vi "Begin.vi"(8 "error in":errorcluster) -> (0 "error out":errorcluster)   [LabVIEW 2020]
doc: "Called before other user functions, this VI is expected to open initial I/O refnums, load in file data, and do all program initialization. Notice that the <B>error out</B> terminal is simply used for data flow. Wiring it to other structures or subVIs ensures that this VI runs first."
uses:
  <vilib>/Rock Robotics/WPI/DriverStation/WPI_DriverStationRobotMode2.ctl
  <vilib>/Rock Robotics/WPI/Joystick/WPI_JoystickDeviceEnum.ctl
  <vilib>/Rock Robotics/SystemInterfaces/i2clib/i2c_bus.ctl
  <vilib>/Rock Robotics/SystemInterfaces/DIO/FPGA_DIOChannel.ctl
  Robot Global Data.vi
  <vilib>/Rock Robotics/Network Tables/NT Write String Array.vi
  <vilib>/Rock Robotics/WPI/ThirdParty/Phoenix-LabVIEW/Motor Controller/Get/CTRE_Phoenix_MotorController_GetSelectedSensorData.vi
  <vilib>/Rock Robotics/WPI/Switch/WPI_SwitchOpenLimit.vi
  <vilib>/Rock Robotics/WPI/Switch/WPI_SwitchOpenCounting.vi
  <vilib>/Rock Robotics/WPI/ThirdParty/Phoenix-LabVIEW/Motor Controller/Get/CTRE_Phoenix_MotorController_IntegratedSensorData_TalonFX.vi
  GlobalAutonVariables.vi
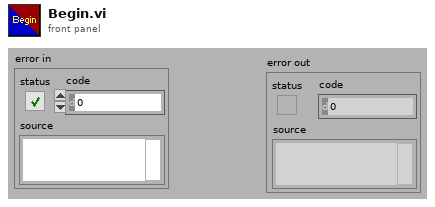
[diagram p1: front panel]
types:
  T1 = typedef "FPGA_DIOChannel.ctl" = enum8{"DIO 0", "DIO 1", "DIO 2", "DIO 3", "DIO 4", "DIO 5", "DIO 6", "DIO 7", "DIO 8", "DIO 9", "DIO MXP 0", "DIO MXP 1", "DIO MXP 2", "DIO MXP 3", "DIO MXP 4", "DIO MXP 5", "DIO MXP 6", "DIO MXP 7", "DIO MXP 8", "DIO MXP 9", "DIO MXP 10", "DIO MXP 11", "DIO MXP 12", "DIO MXP 13", "DIO MXP 14", "DIO MXP 15", "SPI Port CS1", "SPI Port CS2", "SPI Port CS3", "SPI Port MISO", "SPI Port MOSI", "Invalid"}
  T2 = typedef "i2c_bus.ctl" = enum16{"I2C On-Board", "I2C MXP", "Invalid"}
  T3 = typedef "WPI_JoystickDeviceEnum.ctl" = enum16{"USB 0", "USB 1", "USB 2", "USB 3", "USB 4", "USB 5"}
  T4 = typedef "WPI_DriverStationRobotMode2.ctl" = enum16{"Autonomous Disabled", "Autonomous Enabled", "Teleop Disabled", "Teleop Enabled", "Disconnected", "Finish", "Test Disabled", "Test Enabled", "Emergency Stopped"}
  T5 = typedef "WPI_CompressorDevRef.ctl" = cluster{"DevStatus":errorcluster, "Pneumatics Control Module":u8}
  T6 = typedef "WPI_JoystickDevRef.ctl" = cluster{"Device":T3}
  T7 = typedef "WPI_MotorControlDeviceRef.ctl" = cluster{"DeviceStatus":errorcluster, "Type":T8, "PWM":cluster{"PWM Channel":T9, "DeadBand":T10}, "CAN":cluster{"Device Number":u8, "SetOutput VI Ref":variant, "GetOutput VI Ref":variant, "Enable VI Ref":variant, "Disable VI Ref":variant, "Data":variant}, "Invert":bool, "DIO PWM":cluster{"PWM \"Enable\" Channel":T9, "DIOChannel":T1, "PWM Rate":dbl}}
  T8 = typedef "WPI_MotorControlType.ctl" = enum16{"PWM", "CAN", "DIO PWM"}
  T9 = typedef "FPGA_DIOPWMChannel.ctl" = enum8{"PWM 0", "PWM 1", "PWM 2", "PWM 3", "PWM 4", "PWM 5", "PWM 6", "PWM 7", "PWM 8", "PWM 9", "PWM MXP 0", "PWM MXP 1", "PWM MXP 2", "PWM MXP 3", "PWM MXP 4", "PWM MXP 5", "PWM MXP 6", "PWM MXP 7", "PWM MXP 8", "PWM MXP 9", "Invalid"}
  T10 = typedef "WPI_PWMDeadband.ctl" = cluster{"Name":string, "maxPositivePwm":i32, "minPositivePwm":i32, "centerPwm":i32, "maxNegativePwm":i32, "minNegativePwm":i32, "angularRange":u16}
  T11 = typedef "Color Sensor V3 DevRef.ctl" = cluster{"I2CDevRef":T12}
  T12 = typedef "WPI_I2CDevRef.ctl" = cluster{"DevStatus":errorcluster, "Device Address":u8, "Handle":i32, "I2C Bus":T2}
  T13 = typedef "CTRE_PigeonIMU_DeviceRef.ctl" = cluster{"DeviceStatus":errorcluster, "Device Number":u8, "Type":T14, "Device ID":u32, "Handle":u64, "UsageFrame":u32, "Library Path":path}
  T14 = typedef "CTRE_PigeonIMU_ConnectionType.ctl" = u32
  T15 = typedef "CTRE_Phoenix_CANcoder_DeviceRef.ctl" = cluster{"DeviceStatus":errorcluster, "Device Number":u8, "Handle":u64, "UsageFrame":u32, "Library Path":path}
  T16 = typedef "WPI_SwitchDevRef.ctl" = cluster{"DevStatus":errorcluster, "DIO Channel":T1, "CntIndex":T17, "Normally Closed":bool}
  T17 = typedef "FPGA_CounterCtrSystemIndex.ctl" = enum8{"Ctr 0", "Ctr 1", "Ctr 2", "Ctr 3", "Ctr 4", "Ctr 5", "Ctr 6", "Ctr 7", "Invalid"}
  T18 = enum16{"open", "replace", "create", "open or create", "replace or create", "replace or create with confirmation"}
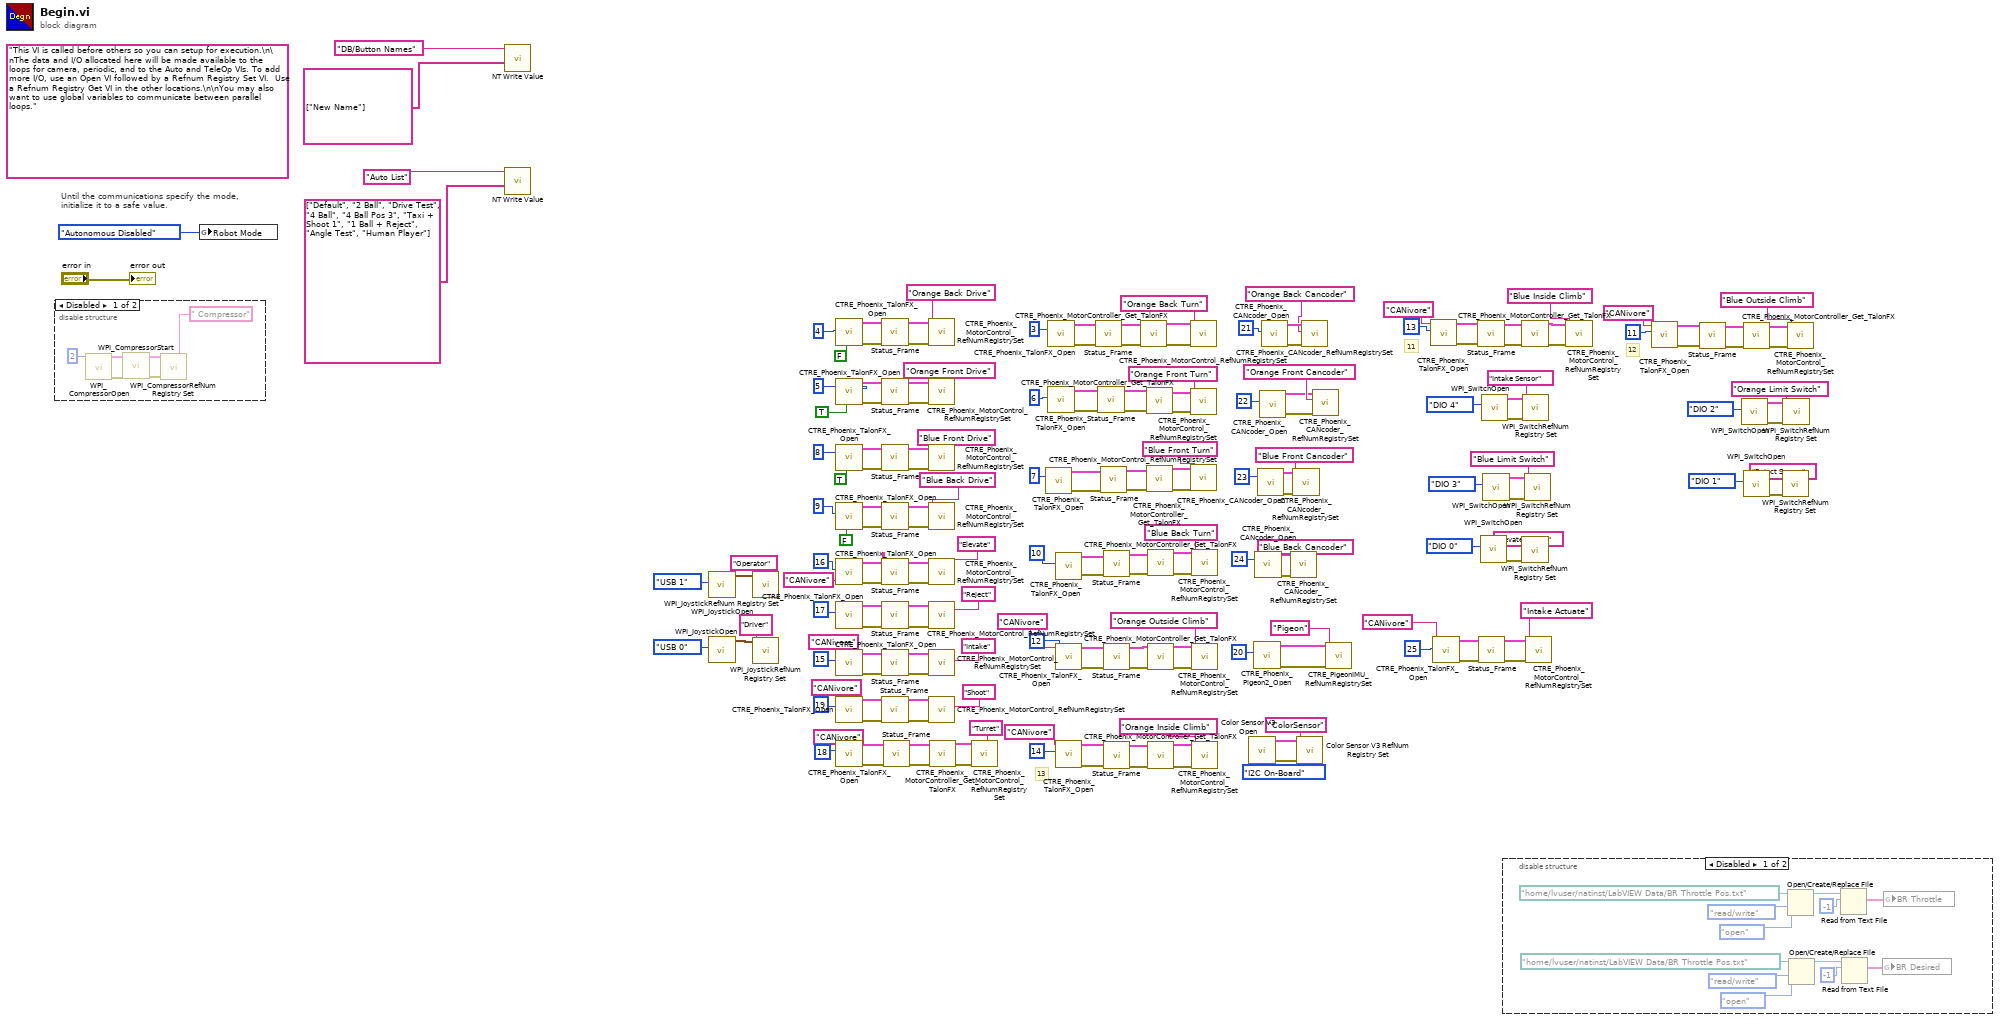
[diagram p0: block diagram]
diagram:
  (unwired) "This VI is called before others so you can setup for execution.\n\nThe data and I/O allocated here will be made available to the loops for camera, periodic, and to the Auto and TeleOp VIs. To add more I/O, use an Open VI followed by a Refnum Registry Set VI.  Use a Refnum Registry Get VI in the other locations.\n\nYou may also want to use global variables to communicate between parallel loops."
  # "13"
  # "12"
  # "11"
  # "Until the communications specify the mode,\ninitialize it to a safe value."
  n1 = disable-structure shown="Disabled" {
    frame Disabled {
      n2 = call <vilib>:"WPI_CompressorOpen.vi"("Pneumatics device (def)"=u8 2) -> ("CompressorDevRef"=w200:T5, "error out"=w201:errorcluster)  [unwired: 13 in]
      n3 = call <vilib>:"WPI_CompressorStart.vi"("error in (no error)"=w201, "CompressorDevRef"=w200) -> ("error out"=w199:errorcluster, "CompressorDevRef"=w198:T5)  [unwired: 8 in]
      n4 = call <vilib>:"WPI_CompressorRefNum Registry Set.vi"("error in (no error)"=w199, "refnum name"=" Compressor", "CompressorDevRef"=w198) -> ()  [unwired: 7 in, 2 out]
    }
    frame Enabled {
    }
  }
  n5 = global write "Robot Global Data.vi" "Robot Mode"(WPI_DriverStationRobotMode2."Autonomous Disabled" ("Robot Mode")) -> ()
  n6 = call-poly <vilib>:"NT Write Value.vi"("String Array"=string[] ["New Name"], "Name"="DB/Button Names") -> ()  [unwired: 9 in, 1 out]
  n7 = call-poly <vilib>:"NT Write Value.vi"("String Array"=string[] ["Default", "2 Ball", "Drive Test", "4 Ball", "4 Ball Pos 3", "Taxi + Shoot 1", "1 Ball + Reject", "Angle Test", "Human Player"], "Name"="Auto List") -> ()  [unwired: 9 in, 1 out]
  n8 = call <vilib>:"WPI_JoystickOpen.vi"("JoystickDevice"=WPI_JoystickDeviceEnum."USB 1") -> ("JoystickDevRef"=w185:T6)  [unwired: 10 in]
  n9 = call <vilib>:"WPI_JoystickOpen.vi"("JoystickDevice"=WPI_JoystickDeviceEnum."USB 0") -> ("JoystickDevRef"=w193:T6)  [unwired: 10 in]
  n10 = call <vilib>:"WPI_JoystickRefNum Registry Set.vi"("refnum name"="Operator", "JoystickDevRef"=w185) -> ()  [unwired: 8 in, 2 out]
  n11 = call <vilib>:"WPI_JoystickRefNum Registry Set.vi"("refnum name"="Driver", "JoystickDevRef"=w193) -> ()  [unwired: 8 in, 2 out]
  n12 = call <vilib>:"CTRE_Phoenix_TalonFX_Open.vi"("Invert"=FALSE, "Device Number"=u8 4) -> ("error out"=w83:errorcluster, "PhoenixMotorControlDevRef"=w84:T7)  [unwired: 8 in]
  n13 = call <vilib>:"CTRE_Phoenix_TalonFX_Open.vi"("Invert"=TRUE, "Device Number"=u8 5) -> ("error out"=w76:errorcluster, "PhoenixMotorControlDevRef"=w75:T7)  [unwired: 8 in]
  n14 = call <vilib>:"CTRE_Phoenix_TalonFX_Open.vi"("Invert"=TRUE, "Device Number"=u8 8) -> ("error out"=w80:errorcluster, "PhoenixMotorControlDevRef"=w77:T7)  [unwired: 8 in]
  n15 = call <vilib>:"CTRE_Phoenix_TalonFX_Open.vi"("Invert"=FALSE, "Device Number"=u8 9) -> ("error out"=w69:errorcluster, "PhoenixMotorControlDevRef"=w72:T7)  [unwired: 8 in]
  n16 = call <vilib>:"CTRE_Phoenix_TalonFX_Open.vi"("Device Number"=u8 16, "CAN Bus"="CANivore") -> ("error out"=w65:errorcluster, "PhoenixMotorControlDevRef"=w68:T7)  [unwired: 8 in]
  n17 = call <vilib>:"CTRE_Phoenix_TalonFX_Open.vi"("Device Number"=u8 17) -> ("error out"=w61:errorcluster, "PhoenixMotorControlDevRef"=w64:T7)  [unwired: 9 in]
  n18 = call <vilib>:"CTRE_Phoenix_TalonFX_Open.vi"("Device Number"=u8 15, "CAN Bus"="CANivore") -> ("error out"=w57:errorcluster, "PhoenixMotorControlDevRef"=w60:T7)  [unwired: 8 in]
  n19 = call <vilib>:"CTRE_Phoenix_TalonFX_Open.vi"("Device Number"=u8 19, "CAN Bus"="CANivore") -> ("error out"=w53:errorcluster, "PhoenixMotorControlDevRef"=w56:T7)  [unwired: 8 in]
  n20 = call <vilib>:"CTRE_Phoenix_TalonFX_Open.vi"("Device Number"=u8 18, "CAN Bus"="CANivore") -> ("error out"=w50:errorcluster, "PhoenixMotorControlDevRef"=w51:T7)  [unwired: 8 in]
  n21 = call "Status_Frame.vi"("error in (no error)"=w83, "Motor Control DevRef"=w84) -> ("error out"=w82:errorcluster, "PhoenixMotorControlDevRef"=w81:T7)  [unwired: 8 in]
  n22 = call "Status_Frame.vi"("error in (no error)"=w76, "Motor Control DevRef"=w75) -> ("error out"=w73:errorcluster, "PhoenixMotorControlDevRef"=w74:T7)  [unwired: 8 in]
  n23 = call "Status_Frame.vi"("error in (no error)"=w80, "Motor Control DevRef"=w77) -> ("error out"=w79:errorcluster, "PhoenixMotorControlDevRef"=w78:T7)  [unwired: 8 in]
  n24 = call "Status_Frame.vi"("error in (no error)"=w69, "Motor Control DevRef"=w72) -> ("error out"=w70:errorcluster, "PhoenixMotorControlDevRef"=w71:T7)  [unwired: 8 in]
  n25 = call "Status_Frame.vi"("error in (no error)"=w65, "Motor Control DevRef"=w68) -> ("error out"=w66:errorcluster, "PhoenixMotorControlDevRef"=w67:T7)  [unwired: 8 in]
  n26 = call "Status_Frame.vi"("error in (no error)"=w61, "Motor Control DevRef"=w64) -> ("error out"=w62:errorcluster, "PhoenixMotorControlDevRef"=w63:T7)  [unwired: 8 in]
  n27 = call "Status_Frame.vi"("error in (no error)"=w57, "Motor Control DevRef"=w60) -> ("error out"=w58:errorcluster, "PhoenixMotorControlDevRef"=w59:T7)  [unwired: 8 in]
  n28 = call "Status_Frame.vi"("error in (no error)"=w53, "Motor Control DevRef"=w56) -> ("error out"=w54:errorcluster, "PhoenixMotorControlDevRef"=w55:T7)  [unwired: 8 in]
  n29 = call "Status_Frame.vi"("error in (no error)"=w50, "Motor Control DevRef"=w51) -> ("error out"=w11:errorcluster, "PhoenixMotorControlDevRef"=w12:T7)  [unwired: 8 in]
  n30 = call <vilib>:"CTRE_Phoenix_MotorControl_RefNumRegistrySet.vi"("error in (no error)"=w82, "refnum name"="Orange Back Drive", "PhoenixMotorControlDevRef"=w81) -> ()  [unwired: 7 in, 2 out]
  n31 = call <vilib>:"CTRE_Phoenix_MotorControl_RefNumRegistrySet.vi"("error in (no error)"=w73, "refnum name"="Orange Front Drive", "PhoenixMotorControlDevRef"=w74) -> ()  [unwired: 7 in, 2 out]
  n32 = call <vilib>:"CTRE_Phoenix_MotorControl_RefNumRegistrySet.vi"("error in (no error)"=w79, "refnum name"="Blue Front Drive", "PhoenixMotorControlDevRef"=w78) -> ()  [unwired: 7 in, 2 out]
  n33 = call <vilib>:"CTRE_Phoenix_MotorControl_RefNumRegistrySet.vi"("error in (no error)"=w70, "refnum name"="Blue Back Drive", "PhoenixMotorControlDevRef"=w71) -> ()  [unwired: 7 in, 2 out]
  n34 = call <vilib>:"CTRE_Phoenix_MotorControl_RefNumRegistrySet.vi"("error in (no error)"=w66, "refnum name"="Elevate", "PhoenixMotorControlDevRef"=w67) -> ()  [unwired: 7 in, 2 out]
  n35 = call <vilib>:"CTRE_Phoenix_MotorControl_RefNumRegistrySet.vi"("error in (no error)"=w62, "refnum name"="Reject", "PhoenixMotorControlDevRef"=w63) -> ()  [unwired: 7 in, 2 out]
  n36 = call <vilib>:"CTRE_Phoenix_MotorControl_RefNumRegistrySet.vi"("error in (no error)"=w58, "refnum name"="Intake", "PhoenixMotorControlDevRef"=w59) -> ()  [unwired: 7 in, 2 out]
  n37 = call <vilib>:"CTRE_Phoenix_MotorControl_RefNumRegistrySet.vi"("error in (no error)"=w54, "refnum name"="Shoot", "PhoenixMotorControlDevRef"=w55) -> ()  [unwired: 7 in, 2 out]
  n38 = call-poly <vilib>:"CTRE_Phoenix_MotorController_Get_TalonFX.vi"("PhoenixMotorControlDevRef"=w12, "error in"=w11) -> ("PhoenixMotorControlDevRef"=w9:T7, "error out"=w10:errorcluster)  [unwired: 9 in, 3 out]
  n39 = call <vilib>:"CTRE_Phoenix_MotorControl_RefNumRegistrySet.vi"("error in (no error)"=w10, "refnum name"="Turret", "PhoenixMotorControlDevRef"=w9) -> ()  [unwired: 7 in, 2 out]
  n40 = call <vilib>:"CTRE_Phoenix_TalonFX_Open.vi"("Device Number"=u8 7) -> ("error out"=w38:errorcluster, "PhoenixMotorControlDevRef"=w41:T7)  [unwired: 9 in]
  n41 = call <vilib>:"CTRE_Phoenix_TalonFX_Open.vi"("Device Number"=u8 3) -> ("error out"=w46:errorcluster, "PhoenixMotorControlDevRef"=w49:T7)  [unwired: 9 in]
  n42 = call <vilib>:"CTRE_Phoenix_TalonFX_Open.vi"("Device Number"=u8 6) -> ("error out"=w42:errorcluster, "PhoenixMotorControlDevRef"=w45:T7)  [unwired: 9 in]
  n43 = call <vilib>:"CTRE_Phoenix_TalonFX_Open.vi"("Device Number"=u8 10) -> ("error out"=w34:errorcluster, "PhoenixMotorControlDevRef"=w35:T7)  [unwired: 9 in]
  n44 = call <vilib>:"CTRE_Phoenix_TalonFX_Open.vi"("Device Number"=u8 12, "CAN Bus"="CANivore") -> ("error out"=w24:errorcluster, "PhoenixMotorControlDevRef"=w25:T7)  [unwired: 8 in]
  n45 = call <vilib>:"CTRE_Phoenix_TalonFX_Open.vi"("Device Number"=u8 14, "CAN Bus"="CANivore") -> ("error out"=w22:errorcluster, "PhoenixMotorControlDevRef"=w23:T7)  [unwired: 8 in]
  n46 = call "Status_Frame.vi"("error in (no error)"=w46, "Motor Control DevRef"=w49) -> ("error out"=w47:errorcluster, "PhoenixMotorControlDevRef"=w48:T7)  [unwired: 8 in]
  n47 = call "Status_Frame.vi"("error in (no error)"=w42, "Motor Control DevRef"=w45) -> ("error out"=w43:errorcluster, "PhoenixMotorControlDevRef"=w44:T7)  [unwired: 8 in]
  n48 = call "Status_Frame.vi"("error in (no error)"=w38, "Motor Control DevRef"=w41) -> ("error out"=w39:errorcluster, "PhoenixMotorControlDevRef"=w40:T7)  [unwired: 8 in]
  n49 = call "Status_Frame.vi"("error in (no error)"=w34, "Motor Control DevRef"=w35) -> ("error out"=w36:errorcluster, "PhoenixMotorControlDevRef"=w37:T7)  [unwired: 8 in]
  n50 = call "Status_Frame.vi"("error in (no error)"=w24, "Motor Control DevRef"=w25) -> ("error out"=w32:errorcluster, "PhoenixMotorControlDevRef"=w33:T7)  [unwired: 8 in]
  n51 = call "Status_Frame.vi"("error in (no error)"=w22, "Motor Control DevRef"=w23) -> ("error out"=w30:errorcluster, "PhoenixMotorControlDevRef"=w31:T7)  [unwired: 8 in]
  n52 = call-poly <vilib>:"CTRE_Phoenix_MotorController_Get_TalonFX.vi"("PhoenixMotorControlDevRef"=w48, "error in"=w47) -> ("PhoenixMotorControlDevRef"=w100:T7, "error out"=w183:errorcluster)  [unwired: 10 in, 2 out]
  n53 = call-poly <vilib>:"CTRE_Phoenix_MotorController_Get_TalonFX.vi"("PhoenixMotorControlDevRef"=w44, "error in"=w43) -> ("PhoenixMotorControlDevRef"=w176:T7, "error out"=w177:errorcluster)  [unwired: 10 in, 2 out]
  n54 = call-poly <vilib>:"CTRE_Phoenix_MotorController_Get_TalonFX.vi"("PhoenixMotorControlDevRef"=w40, "error in"=w39) -> ("PhoenixMotorControlDevRef"=w106:T7, "error out"=w101:errorcluster)  [unwired: 10 in, 2 out]
  n55 = call-poly <vilib>:"CTRE_Phoenix_MotorController_Get_TalonFX.vi"("PhoenixMotorControlDevRef"=w37, "error in"=w36) -> ("PhoenixMotorControlDevRef"=w102:T7, "error out"=w164:errorcluster)  [unwired: 10 in, 2 out]
  n56 = call-poly <vilib>:"CTRE_Phoenix_MotorController_Get_TalonFX.vi"("PhoenixMotorControlDevRef"=w33, "error in"=w32) -> ("PhoenixMotorControlDevRef"=w103:T7, "error out"=w120:errorcluster)  [unwired: 10 in, 2 out]
  n57 = call-poly <vilib>:"CTRE_Phoenix_MotorController_Get_TalonFX.vi"("PhoenixMotorControlDevRef"=w31, "error in"=w30) -> ("PhoenixMotorControlDevRef"=w105:T7, "error out"=w117:errorcluster)  [unwired: 10 in, 2 out]
  n58 = call <vilib>:"CTRE_Phoenix_MotorControl_RefNumRegistrySet.vi"("error in (no error)"=w183, "refnum name"="Orange Back Turn", "PhoenixMotorControlDevRef"=w100) -> ()  [unwired: 7 in, 2 out]
  n59 = call <vilib>:"CTRE_Phoenix_MotorControl_RefNumRegistrySet.vi"("error in (no error)"=w177, "refnum name"="Orange Front Turn", "PhoenixMotorControlDevRef"=w176) -> ()  [unwired: 7 in, 2 out]
  n60 = call <vilib>:"CTRE_Phoenix_MotorControl_RefNumRegistrySet.vi"("error in (no error)"=w101, "refnum name"="Blue Front Turn", "PhoenixMotorControlDevRef"=w106) -> ()  [unwired: 7 in, 2 out]
  n61 = call <vilib>:"CTRE_Phoenix_MotorControl_RefNumRegistrySet.vi"("error in (no error)"=w164, "refnum name"="Blue Back Turn", "PhoenixMotorControlDevRef"=w102) -> ()  [unwired: 7 in, 2 out]
  n62 = call <vilib>:"CTRE_Phoenix_MotorControl_RefNumRegistrySet.vi"("error in (no error)"=w120, "refnum name"="Orange Outside Climb", "PhoenixMotorControlDevRef"=w103) -> ()  [unwired: 7 in, 2 out]
  n63 = call <vilib>:"CTRE_Phoenix_MotorControl_RefNumRegistrySet.vi"("error in (no error)"=w117, "refnum name"="Orange Inside Climb", "PhoenixMotorControlDevRef"=w105) -> ()  [unwired: 7 in, 2 out]
  n64 = call <vilib>:"Color Sensor V3 Open.vi"("I2C Bus"=i2c_bus."I2C On-Board") -> ("error out"=w148:errorcluster, "ColorSensorDevRef"=w147:T11)  [unwired: 9 in]
  n65 = call <vilib>:"CTRE_Phoenix_Pigeon2_Open.vi"("Device Number"=u8 20) -> ("error out"=w13:errorcluster, "PigeonIMUDevRef"=w14:T13)  [unwired: 9 in]
  n66 = call <vilib>:"CTRE_Phoenix_CANcoder_Open.vi"("Device Number"=u8 24) -> ("error out"=w95:errorcluster, "CTRE_CANcoder_DeviceRef"=w96:T15)  [unwired: 9 in]
  n67 = call <vilib>:"CTRE_Phoenix_CANcoder_Open.vi"("Device Number"=u8 23) -> ("error out"=w97:errorcluster, "CTRE_CANcoder_DeviceRef"=w98:T15)  [unwired: 9 in]
  n68 = call <vilib>:"CTRE_Phoenix_CANcoder_Open.vi"("Device Number"=u8 22) -> ("error out"=w94:errorcluster, "CTRE_CANcoder_DeviceRef"=w93:T15)  [unwired: 9 in]
  n69 = call <vilib>:"CTRE_Phoenix_CANcoder_Open.vi"("Device Number"=u8 21) -> ("error out"=w16:errorcluster, "CTRE_CANcoder_DeviceRef"=w17:T15)  [unwired: 9 in]
  n70 = call <vilib>:"CTRE_Phoenix_CANcoder_RefNumRegistrySet.vi"("error in (no error)"=w95, "refnum name"="Blue Back Cancoder", "CTRE_CANcoder_DeviceRef"=w96) -> ()  [unwired: 7 in, 2 out]
  n71 = call <vilib>:"CTRE_Phoenix_CANcoder_RefNumRegistrySet.vi"("error in (no error)"=w97, "refnum name"="Blue Front Cancoder", "CTRE_CANcoder_DeviceRef"=w98) -> ()  [unwired: 7 in, 2 out]
  n72 = call <vilib>:"Color Sensor V3 RefNum Registry Set.vi"("error in (no error)"=w148, "refnum name"="ColorSensor", "ColorSensorDevRef"=w147) -> ()  [unwired: 7 in, 2 out]
  n73 = call <vilib>:"CTRE_Phoenix_CANcoder_RefNumRegistrySet.vi"("error in (no error)"=w16, "refnum name"="Orange Back Cancoder", "CTRE_CANcoder_DeviceRef"=w17) -> ()  [unwired: 7 in, 2 out]
  n74 = call <vilib>:"CTRE_Phoenix_CANcoder_RefNumRegistrySet.vi"("error in (no error)"=w94, "refnum name"="Orange Front Cancoder", "CTRE_CANcoder_DeviceRef"=w93) -> ()  [unwired: 7 in, 2 out]
  n75 = call <vilib>:"CTRE_PigeonIMU_RefNumRegistrySet.vi"("error in (no error)"=w13, "refnum name"="Pigeon", "PigeonIMUDevRef"=w14) -> ()  [unwired: 7 in, 2 out]
  n76 = call <vilib>:"CTRE_Phoenix_TalonFX_Open.vi"("Device Number"=u8 13, "CAN Bus"="CANivore") -> ("error out"=w18:errorcluster, "PhoenixMotorControlDevRef"=w19:T7)  [unwired: 8 in]
  n77 = call <vilib>:"CTRE_Phoenix_TalonFX_Open.vi"("Device Number"=u8 25, "CAN Bus"="CANivore") -> ("error out"=w4:errorcluster, "PhoenixMotorControlDevRef"=w6:T7)  [unwired: 8 in]
  n78 = call "Status_Frame.vi"("error in (no error)"=w18, "Motor Control DevRef"=w19) -> ("error out"=w26:errorcluster, "PhoenixMotorControlDevRef"=w27:T7)  [unwired: 8 in]
  n79 = call "Status_Frame.vi"("error in (no error)"=w4, "Motor Control DevRef"=w6) -> ("error out"=w3:errorcluster, "PhoenixMotorControlDevRef"=w5:T7)  [unwired: 8 in]
  n80 = call-poly <vilib>:"WPI_SwitchOpen.vi"("DIO Channel"=FPGA_DIOChannel."DIO 0") -> ("error out"=w144:errorcluster, "SwitchDevRef"=w143:T16)  [unwired: 9 in]
  n81 = call-poly <vilib>:"WPI_SwitchOpen.vi"("DIO Channel"=FPGA_DIOChannel."DIO 4") -> ("error out"=w124:errorcluster, "SwitchDevRef"=w123:T16)  [unwired: 9 in]
  n82 = call-poly <vilib>:"WPI_SwitchOpen.vi"("DIO Channel"=FPGA_DIOChannel."DIO 3") -> ("error out"=w128:errorcluster, "SwitchDevRef"=w127:T16)  [unwired: 9 in]
  n83 = disable-structure shown="Disabled" {
    frame Disabled {
      n84 = Open/Create/Replace File(file path (use dialog)=path "/home/lvuser/natinst/LabVIEW Data/BR Throttle Pos.txt", operation (0:open)=T18."open", access (0:read/write)=enum16{"read/write", "read-only", "write-only"}."read/write") -> (refnum out=w210:refnum<file>)  [unwired: 3 in, 2 out]
      n85 = Open/Create/Replace File(file path (use dialog)=path "/home/lvuser/natinst/LabVIEW Data/BR Throttle Pos.txt", operation (0:open)=T18."open", access (0:read/write)=enum16{"read/write", "read-only", "write-only"}."read/write") -> (refnum out=w205:refnum<file>)  [unwired: 3 in, 2 out]
      n86 = Read from Text File(file (use dialog)=w210, count=-1) -> (text=w203:string[])  [unwired: 2 in, 3 out]
      n87 = Read from Text File(file (use dialog)=w205, count=-1) -> (text=w202:string[])  [unwired: 2 in, 3 out]
      n88 = global write "GlobalAutonVariables.vi" "BR Desired"(w202) -> ()
      n89 = global write "GlobalAutonVariables.vi" "BR Throttle"(w203) -> ()
    }
    frame Enabled {
    }
  }
  n90 = call-poly <vilib>:"CTRE_Phoenix_MotorController_Get_TalonFX.vi"("PhoenixMotorControlDevRef"=w27, "error in"=w26) -> ("PhoenixMotorControlDevRef"=w109:T7, "error out"=w110:errorcluster)  [unwired: 10 in, 2 out]
  n91 = call <vilib>:"WPI_SwitchRefNum Registry Set.vi"("error in (no error)"=w144, "refnum name"="Elevate Sensor", "SwitchDevRef"=w143) -> ()  [unwired: 7 in, 2 out]
  n92 = call <vilib>:"WPI_SwitchRefNum Registry Set.vi"("error in (no error)"=w124, "refnum name"="Intake Sensor", "SwitchDevRef"=w123) -> ()  [unwired: 7 in, 2 out]
  n93 = call <vilib>:"WPI_SwitchRefNum Registry Set.vi"("error in (no error)"=w128, "refnum name"="Blue Limit Switch", "SwitchDevRef"=w127) -> ()  [unwired: 7 in, 2 out]
  n94 = call <vilib>:"CTRE_Phoenix_MotorControl_RefNumRegistrySet.vi"("error in (no error)"=w3, "refnum name"="Intake Actuate", "PhoenixMotorControlDevRef"=w5) -> ()  [unwired: 7 in, 2 out]
  n95 = call <vilib>:"CTRE_Phoenix_MotorControl_RefNumRegistrySet.vi"("error in (no error)"=w110, "refnum name"="Blue Inside Climb", "PhoenixMotorControlDevRef"=w109) -> ()  [unwired: 7 in, 2 out]
  n96 = call <vilib>:"CTRE_Phoenix_TalonFX_Open.vi"("Device Number"=u8 11, "CAN Bus"="CANivore") -> ("error out"=w20:errorcluster, "PhoenixMotorControlDevRef"=w21:T7)  [unwired: 8 in]
  n97 = call "Status_Frame.vi"("error in (no error)"=w20, "Motor Control DevRef"=w21) -> ("error out"=w28:errorcluster, "PhoenixMotorControlDevRef"=w29:T7)  [unwired: 8 in]
  n98 = call-poly <vilib>:"WPI_SwitchOpen.vi"("DIO Channel"=FPGA_DIOChannel."DIO 2") -> ("error out"=w132:errorcluster, "SwitchDevRef"=w131:T16)  [unwired: 9 in]
  n99 = call-poly <vilib>:"CTRE_Phoenix_MotorController_Get_TalonFX.vi"("PhoenixMotorControlDevRef"=w29, "error in"=w28) -> ("PhoenixMotorControlDevRef"=w113:T7, "error out"=w114:errorcluster)  [unwired: 10 in, 2 out]
  n100 = call-poly <vilib>:"WPI_SwitchOpen.vi"("DIO Channel"=FPGA_DIOChannel."DIO 1") -> ("error out"=w140:errorcluster, "SwitchDevRef"=w139:T16)  [unwired: 9 in]
  n101 = call <vilib>:"WPI_SwitchRefNum Registry Set.vi"("error in (no error)"=w140, "refnum name"="Reject Sensor", "SwitchDevRef"=w139) -> ()  [unwired: 7 in, 2 out]
  n102 = call <vilib>:"WPI_SwitchRefNum Registry Set.vi"("error in (no error)"=w132, "refnum name"="Orange Limit Switch", "SwitchDevRef"=w131) -> ()  [unwired: 7 in, 2 out]
  n103 = call <vilib>:"CTRE_Phoenix_MotorControl_RefNumRegistrySet.vi"("error in (no error)"=w114, "refnum name"="Blue Outside Climb", "PhoenixMotorControlDevRef"=w113) -> ()  [unwired: 7 in, 2 out]
  "error out" <- "error in"
